vi "335 Read and Compressor auto control(SubVI).vi"(6 "压缩机自动停机":bool, 9 "自动控制":bool, 10 "数值":i32, 11 "Instrument":T1 {"Input (0:A)" items=["A", "B"]; "Instrument Type" items=["PPMS", "VersaLab", "DynaCool", "SVSM", "Lakeshore335", "PPMS-Rotate"]; "Heater Output (1:1)" items=["1"=1, "2"=2]}) -> (3 "簇":T4 {"?" items=["Unknow", "Stable", "Following Warm", "Following Cold", "Unfollowing"]})   [LabVIEW 2019]
uses:
  335 state.ctl
  Instrument.ctl
  <vilib>/NI/Modbus Library/API/Master/Modbus Master.lvclass
  lib/QDInstrument.dll
  lib/Lake Shore 335/Lake Shore 335.lvlib
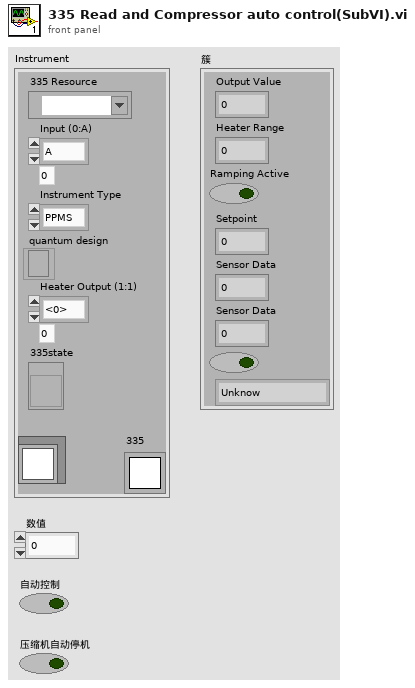
[diagram p1: front panel]
types:
  T1 = typedef "Instrument.ctl" = cluster{"335 Resource":refnum<visa-resource-name>, "Input (0:A)":u16, "Instrument Type":i32, "quantum design":refnum<k24>, "Heater Output (1:1)":u16, "335state":refnum<vi>, "semaphore":T2, "TCP master instance":refnum<class "Modbus Master.lvclass">}
  T2 = typedef "Semaphore RefNum" = refnum<k1>
  T3 = typedef "335 state.ctl" = u16
  T4 = cluster{"Output Value":dbl, "Heater Range ":u16, "Ramping Active":bool, "Setpoint":dbl, "Sensor Data":dbl, "Sensor Data":dbl, bool, T3}
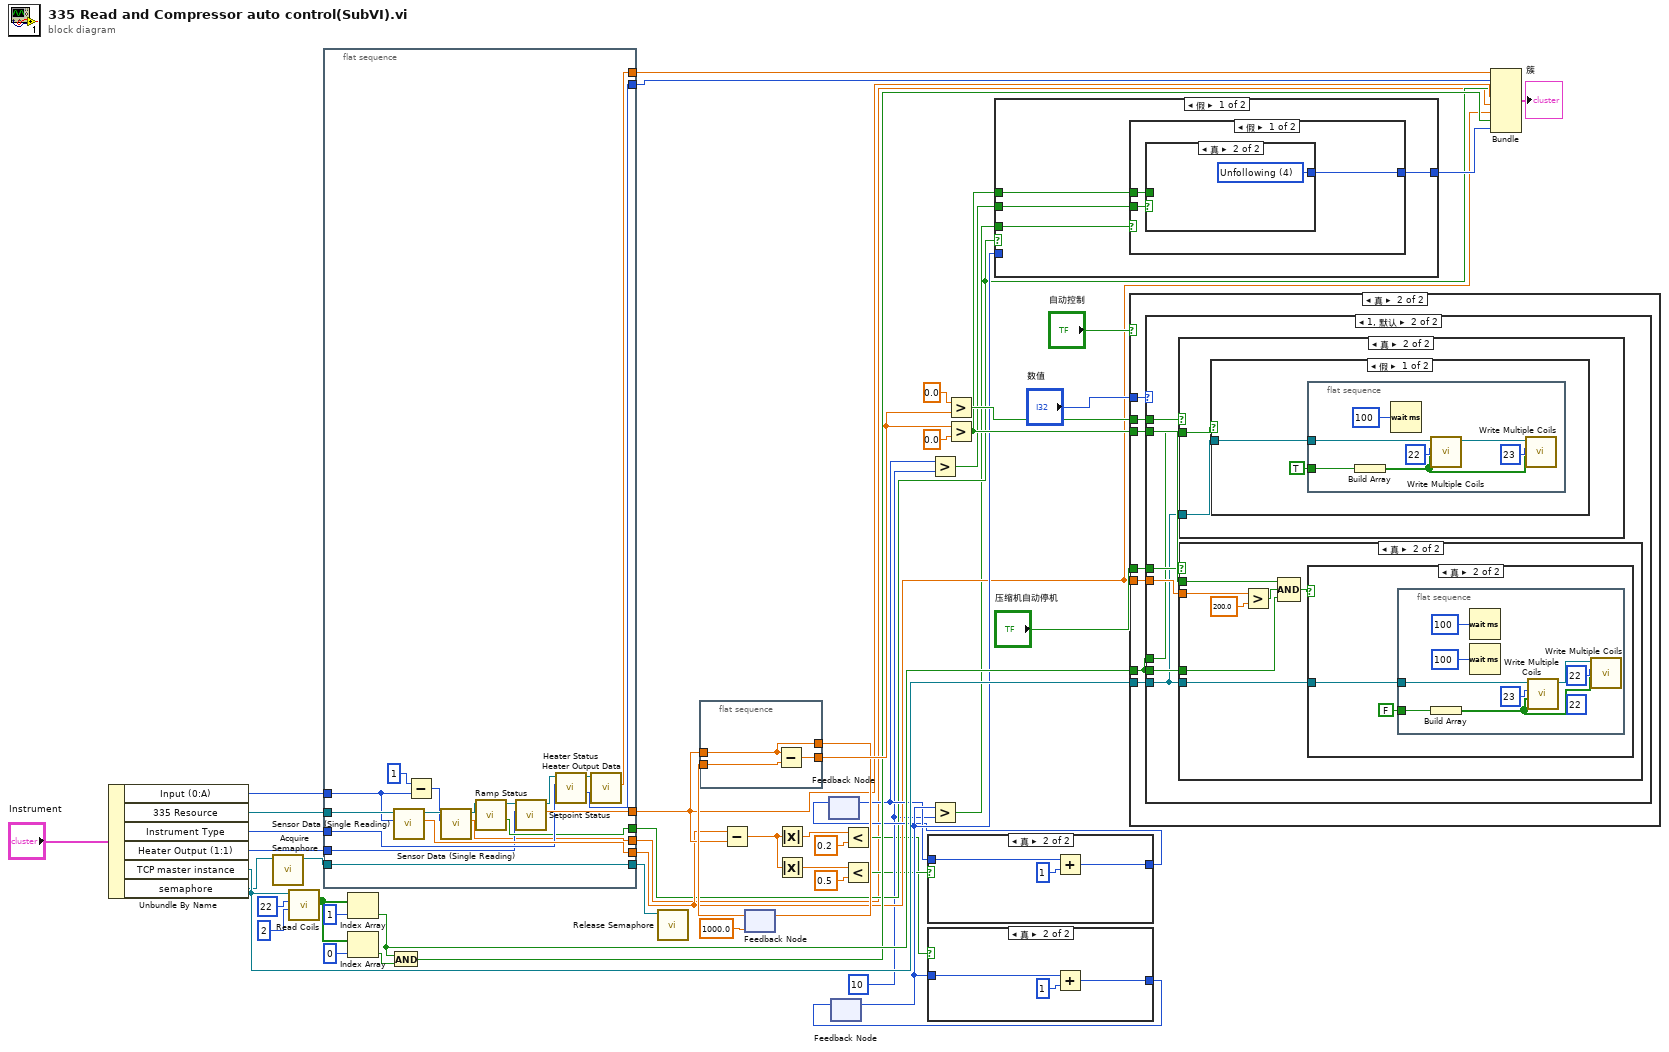
[diagram p0: block diagram]
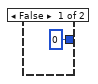
[diagram p8: hidden frame]
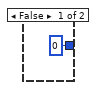
[diagram p9: hidden frame]
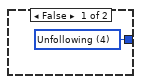
[diagram p10: hidden frame]
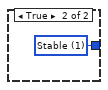
[diagram p11: hidden frame]
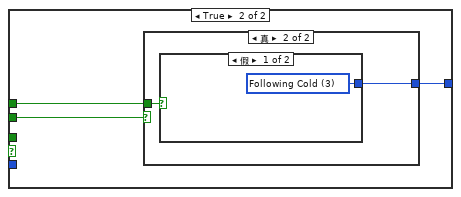
[diagram p12: hidden frame]
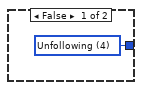
[diagram p13: hidden frame]
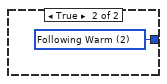
[diagram p14: hidden frame]
diagram:
  w21 = 10 ("y")
  n1 = Unbundle By Name("Instrument") -> ("Input (0:A)"=w7:u16, "335 Resource"=w2:refnum<visa-resource-name>, "Instrument Type"=w3:i32, "Heater Output (1:1)"=w6:u16, "TCP master instance"=w48:refnum<class "Modbus Master.lvclass">, "semaphore"=w30:T2)
  n2 = call <vilib>:"Acquire Semaphore.vi"("semaphore"=w30) -> ("semaphore out"=w4:T2)  [unwired: 4 in, 2 out]
  n3 = call-dynamic "Read Coils.vi"("number of inputs"=u16 2, "starting address"=u16 22, "Modbus master in"=w48) -> ("coils"=w35:bool[])  [unwired: 6 in, 2 out]
  n4 = flat-sequence {
    tunnel: [w68] -> w36
    tunnel: w2 -> [w66]
    tunnel: [w63] -> w25
    tunnel: w3 -> [w62]
    tunnel: w4 -> [w61]
    tunnel: [w61] -> w5
    tunnel: [w60] -> w9
    tunnel: [w59] -> w8
    tunnel: [w58] -> w24
    tunnel: w6 -> [w57]
    tunnel: w7 -> [w56]
    tunnel: [w51] -> w10
    frame #0 {
      n5 = call "Sensor Data (Single Reading).vi"("Input (0:A)"=w56, "VISA resource name"=w66) -> ("Sensor Data"=w63:dbl, "VISA resource name out"=w54:refnum<visa-resource-name>)  [unwired: 7 in, 1 out]
      n6 = Subtract(x=u16 1, y=w56) -> (x-y=w52:u16)
      n7 = call "Sensor Data (Single Reading).vi"("Input (0:A)"=w52, "VISA resource name"=w54) -> ("Sensor Data"=w51:dbl, "VISA resource name out"=w53:refnum<visa-resource-name>)  [unwired: 7 in, 1 out]
      n8 = call "Ramp Status.vi"("VISA resource name"=w53) -> ("Ramping Active"=w58:bool, "VISA resource name out"=w67:refnum<visa-resource-name>)  [unwired: 6 in, 3 out]
      n9 = call "Setpoint Status.vi"("Output (1:1)"=w57, "VISA resource name"=w67) -> ("Setpoint"=w68:dbl, "VISA resource name out"=w65:refnum<visa-resource-name>)  [unwired: 7 in, 1 out]
      n10 = call "Heater Status.vi"("Heater Output (1:1)"=w62, "VISA resource name"=w65) -> ("Heater Range"=w60:u16, "VISA resource name out"=w64:refnum<visa-resource-name>)  [unwired: 5 in, 3 out]
      n11 = call "Heater Output Data.vi"("VISA resource name"=w64) -> ("Output Value"=w59:dbl)  [unwired: 8 in, 2 out]
    }
  }
  n12 = Index Array(array=w35, index=1) -> (element=w47:bool)
  n13 = Index Array(array=w35, index=0) -> (element=w31:bool)
  n14 = And(x=w47, y=w31) -> (x .and. y?=w32:bool)
  n15 = call <vilib>:"Release Semaphore.vi"("semaphore"=w5) -> ()  [unwired: 5 in, 2 out]
  n16 = flat-sequence {
    tunnel: w36 -> [w71]
    tunnel: [w71] -> w37
    tunnel: w38 -> [w70]
    tunnel: [w69] -> w45
    frame #0 {
      n17 = Subtract(x=w71, y=w70) -> (x-y=w69:dbl)
    }
  }
  n18 = Subtract(x=w25, y=w36) -> (x-y=w19:dbl)
  n19 = feedback #1(1000.0 ("Setpoint")) -> (w38:dbl)
  n20 = feedback-in #1(w37) -> ()
  n21 = Absolute Value(x=w19) -> (abs(x)=w16:dbl)
  n22 = Absolute Value(x=w19) -> (abs(x)=w17:dbl)
  n23 = feedback #2() -> (w27:i32)  [unwired: 1 in]
  n24 = feedback #3() -> (w29:i32)  [unwired: 1 in]
  n25 = Less?(x=w16, y=0.2) -> (x < y?=w15:bool)
  n26 = Less?(x=w17, y=0.5) -> (x < y?=w20:bool)
  n27 = case shown="真" w20 {
    tunnel: w27 -> [_ w75]
    tunnel: [0 w73] -> w26
    frame False {
    }
    frame True {
      n28 = Add(x=w75, y=1) -> (x+y=w73:i32)
    }
  }
  n29 = feedback-in #2(w26) -> ()
  n30 = case shown="真" w15 {
    tunnel: w29 -> [_ w79]
    tunnel: [0 w77] -> w28
    frame False {
    }
    frame True {
      n31 = Add(x=w79, y=1) -> (x+y=w77:i32)
    }
  }
  n32 = feedback-in #3(w28) -> ()
  n33 = Greater?(x=w27, y=w21) -> (0:w23:bool)
  n34 = Greater?(x=w29, y=w21) -> (0:w22:bool)
  n35 = Greater?(x=0.0, y=w45) -> (0:w46:bool)
  n36 = Greater?(x=w45, y=0.0) -> (0:w42:bool)
  n37 = case shown="假" w24 {
    tunnel: w29 -> [_ _]
    tunnel: w22 -> [w83 _]
    tunnel: w23 -> [w82 w92]
    tunnel: [w81 w91] -> w41
    tunnel: w42 -> [w80 w90]
    frame False {
      n38 = case shown="假" w83 {
        tunnel: [w85 w89] -> w81
        tunnel: w82 -> [w86 _]
        tunnel: w80 -> [w84 _]
        frame False {
          n39 = case shown="真" w86 {
            tunnel: [w87 w88] -> w85
            tunnel: w84 -> [_ _]
            frame False {
              w87 = T3 4 items=["Unknow", "Stable", "Following Warm", "Following Cold", "Unfollowing"]
            }
            frame True {
              w88 = T3 4 items=["Unknow", "Stable", "Following Warm", "Following Cold", "Unfollowing"]
            }
          }
        }
        frame True {
          w89 = T3 1 items=["Unknow", "Stable", "Following Warm", "Following Cold", "Unfollowing"]
        }
      }
    }
    frame True {
      n40 = case shown="真" w92 {
        tunnel: [w93 w94] -> w91
        tunnel: w90 -> [_ w95]
        frame False {
          w93 = T3 4 items=["Unknow", "Stable", "Following Warm", "Following Cold", "Unfollowing"]
        }
        frame True {
          n41 = case shown="假" w95 {
            tunnel: [w96 w97] -> w94
            frame False {
              w96 = T3 3 items=["Unknow", "Stable", "Following Warm", "Following Cold", "Unfollowing"]
            }
            frame True {
              w97 = T3 2 items=["Unknow", "Stable", "Following Warm", "Following Cold", "Unfollowing"]
            }
          }
        }
      }
    }
  }
  n42 = case shown="真" "自动控制" {
    tunnel: w25 -> [_ w104]
    tunnel: w42 -> [_ w103]
    tunnel: "压缩机自动停机" -> [_ w102]
    tunnel: "数值" -> [_ w101]
    tunnel: w46 -> [_ w100]
    tunnel: w47 -> [_ w99]
    tunnel: w48 -> [_ w98]
    frame False {
    }
    frame True {
      n43 = case shown="1, 默认" w101 {
        tunnel: w104 -> [_ w111]
        tunnel: w103 -> [_ w110]
        tunnel: w99 -> [_ w109]
        tunnel: w102 -> [_ w108]
        tunnel: w100 -> [_ w107]
        tunnel: w99 -> [_ w106]
        tunnel: w98 -> [_ w105]
        frame 0 {
        }
        frame 1, Default {
          n44 = case shown="真" w107 {
            tunnel: w106 -> [_ w113]
            tunnel: w105 -> [_ w112]
            frame False {
            }
            frame True {
              n45 = case shown="假" w113 {
                tunnel: w112 -> [w114 _]
                frame False {
                  n46 = flat-sequence {
                    tunnel: TRUE -> [w118]
                    tunnel: w114 -> [w121]
                    frame #0 {
                      n47 = Build Array(w118) -> (w117:bool[])
                      n48 = Wait (ms)(milliseconds to wait=u32 100 ("等待时间（毫秒）")) -> ()  [unwired: 1 out]
                      n49 = call-dynamic "Write Multiple Coils.vi"("coils to write"=w117, "starting address"=u16 22, "Modbus master in"=w121) -> ("Modbus master out"=w119:refnum<class "Modbus Master.lvclass">)  [unwired: 7 in, 1 out]
                      n50 = call-dynamic "Write Multiple Coils.vi"("coils to write"=w117, "starting address"=u16 23, "Modbus master in"=w119) -> ()  [unwired: 7 in, 2 out]
                    }
                  }
                }
                frame True {
                }
              }
            }
          }
          n51 = case shown="真" w108 {
            tunnel: w111 -> [_ w129]
            tunnel: w110 -> [_ w127]
            tunnel: w109 -> [_ w126]
            tunnel: w105 -> [_ w123]
            frame False {
            }
            frame True {
              n52 = Greater?(x=w129, y=200.0) -> (0:w125:bool)
              n53 = Compound Arithmetic op=AND ("复合运算")(w127, w125, w126) -> (w124:bool)
              n54 = case shown="真" w124 {
                tunnel: w123 -> [_ w130]
                frame False {
                }
                frame True {
                  n55 = flat-sequence {
                    tunnel: FALSE -> [w135]
                    tunnel: w130 -> [w134]
                    frame #0 {
                      (unwired) u16 22 ("starting address")
                      n56 = Build Array(w135) -> (w132:bool[])
                      n57 = Wait (ms)(milliseconds to wait=u32 100 ("等待时间（毫秒）")) -> ()  [unwired: 1 out]
                      n58 = Wait (ms)(milliseconds to wait=u32 100 ("等待时间（毫秒）")) -> ()  [unwired: 1 out]
                      n59 = call-dynamic "Write Multiple Coils.vi"("coils to write"=w132, "starting address"=u16 23, "Modbus master in"=w134) -> ("Modbus master out"=w133:refnum<class "Modbus Master.lvclass">)  [unwired: 7 in, 1 out]
                      n60 = call-dynamic "Write Multiple Coils.vi"("coils to write"=w132, "starting address"=u16 22, "Modbus master in"=w133) -> ()  [unwired: 7 in, 2 out]
                    }
                  }
                }
              }
            }
          }
        }
      }
    }
  }
  n61 = Bundle("Output Value"=w8, "Heater Range"=w9, "Ramping Active"=w24, "Setpoint"=w36, "Sensor Data"=w10, "Sensor Data"=w25, w32, w41) -> (→"簇":T4)  [unwired: 1 in]
